vi "Deinitialize TDK 20-38.vi"(8 "error":errorcluster, 11 "VISA name":refnum<visa-resource-name>) -> (0 "error out":errorcluster)   [LabVIEW 2023, in "TDK20-38 API.lvlib"]
uses:
  TDK20-38 API.lvlib
  <userlib>/TDK-Lambda GEN LAN Series/TDK-Lambda GEN LAN Series.lvlib
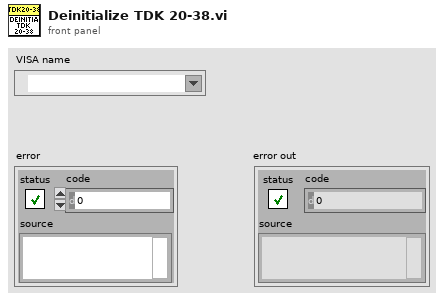
[diagram p1: front panel]
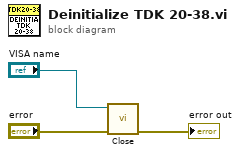
[diagram p0: block diagram]
diagram:
  n1 = call "Close.vi"("error"="error", "VISA name"="VISA name") -> ("error out"=→"error out":errorcluster)  [unwired: 9 in]
